vi "TimerDRV.vi"(8 "error in (no error)":errorcluster, 11 "TimerDRV in":refnum<class "TimerDRV.lvclass">) -> (0 "error out":errorcluster, 3 "TimerDRV out":refnum<class "TimerDRV.lvclass">)   [LabVIEW 2019, in "TimingDRV Engine.lvlib" / "TimerDRV.lvclass"]
uses:
  TimerDRV.lvclass
  TimerDRV.lvclass/TimerDRV.ctl
  <vilib>/Platform/TimedLoop/XDataNode/timing_clust.ctl
  <vilib>/Platform/TimedLoop/XDataNode/nitl_modes.ctl
  <vilib>/Platform/TimedLoop/XDataNode/wakeup.ctl
  TypeDefs/Command.ctl
  <vilib>/platform/TimedLoop/XDataNode/XDataNode.xnode
  <vilib>/Platform/TimedLoop/XDataNode/XDNodeRunTimeDep.lvlib
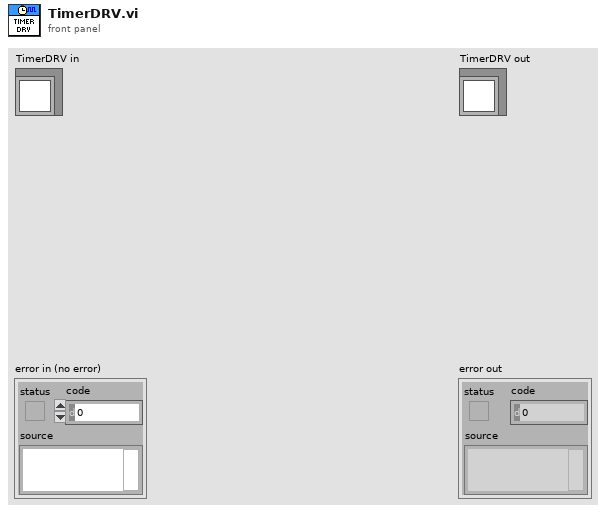
[diagram p1: front panel]
types:
  T1 = typedef "XDNodeRunTimeDep.lvlib/timing_clust.ctl" = cluster{"Expected End [f-1]":u64, "Actual End [f-1]":u64, "Finished Late? [f-1]":bool, "Expected End [i-1]":u64, "Actual End [i-1]":u64, "Finished Late? [i-1]":bool, "Expected Start [i]":u64, "Actual Start [i]":u64, "Expected Start [f]":u64, "Actual Start [f]":u64, "Source Name":string, "Structure Name":string, "Period":i64, "Deadline":i64, "Offset":i64, "Start":i64, "Priority":i32, "Timeout":i32, "Mode":T2, "Wakeup Reason":T3, "Error":errorcluster, "Source Type":string, "Secondary Source Type":string, "Global End Time":u64, "Global Start Time":u64, "Frame Duration":u64, "Iteration Duration":u64, "Assigned CPU":i32, "I/O Scan Engine Mode":u32}
  T2 = typedef "XDNodeRunTimeDep.lvlib/nitl_modes.ctl" = enum32{"No Change", "Process missed periods, maintain original phase", "Discard missed periods, maintain original phase", "Process missed periods, ignore original phase", "Discard missed periods, ignore original phase"}
  T3 = typedef "XDNodeRunTimeDep.lvlib/wakeup.ctl" = enum32{"Normal", "Aborted", "Asynchronous wakeup", "Timing source error", "Timed loop error", "Timeout"}
  T4 = typedef "TimingDRV Engine.lvlib/TimerDRV.lvclass/Command.ctl" = enum16{"Shutdown", "Update Execution Frequency", "Initialize"}
  T5 = typedef "TimingDRV Engine.lvlib/TimerDRV.lvclass/Target Type.ctl" = enum16{"PharLap", "VxWorks", "Windows", "Linux_32_ARM", "Linux_x64"}
  T6 = typedef "TimingDRV Engine.lvlib/TimerDRV.lvclass/Command Package.ctl" = cluster{"Command":T4, "Command Data":variant}
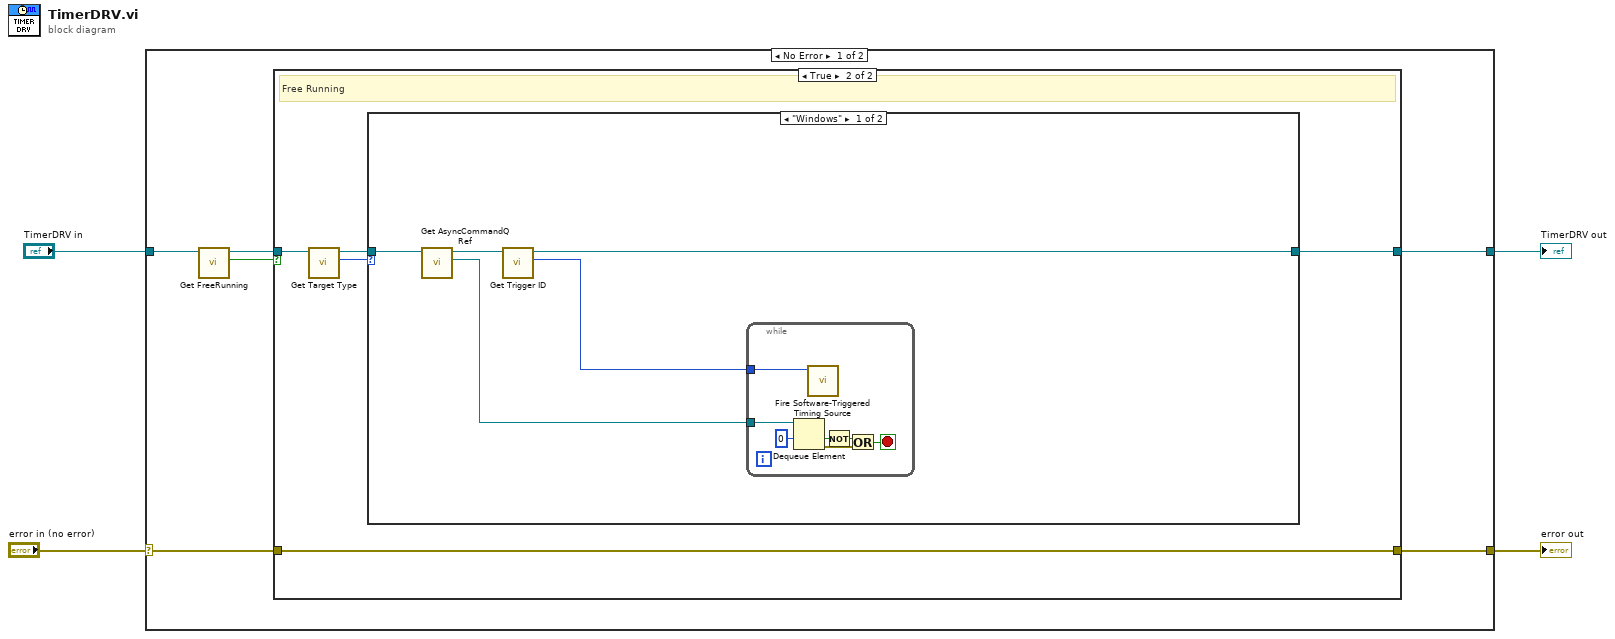
[diagram p0: block diagram]
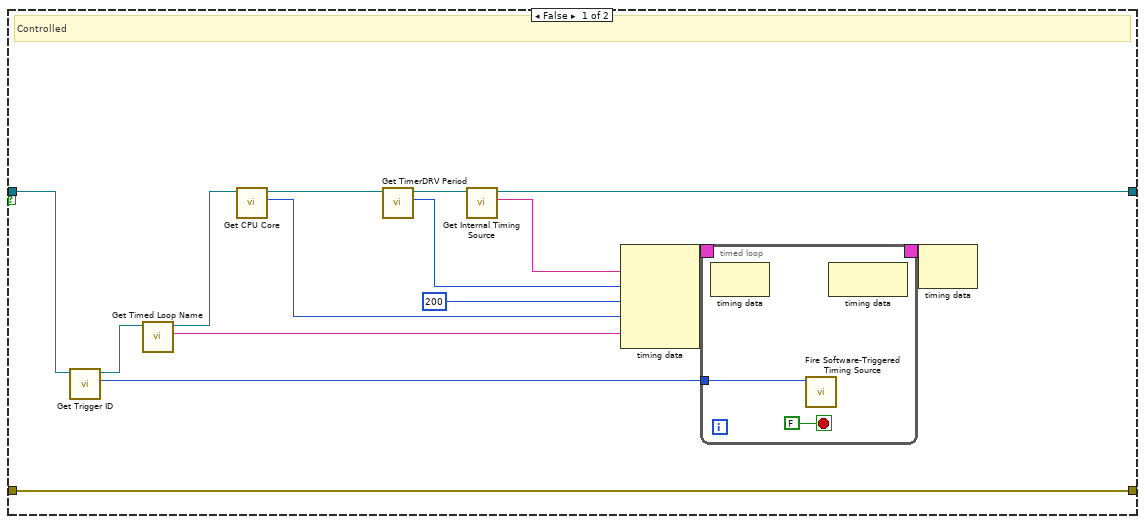
[diagram p2: hidden frame]
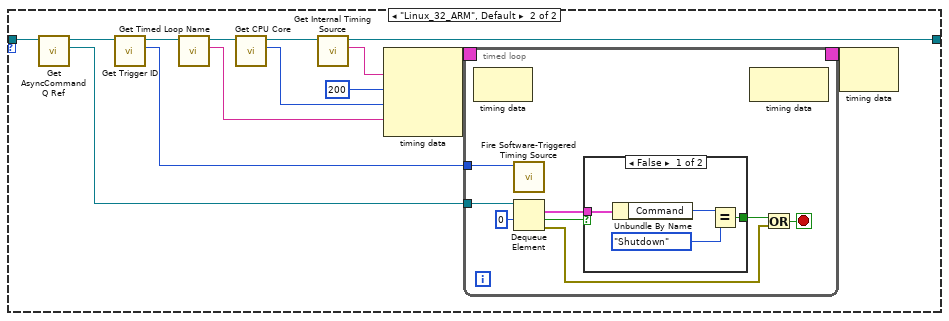
[diagram p3: hidden frame]
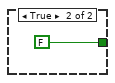
[diagram p4: hidden frame]
diagram:
  n1 = case shown="No Error" "error in (no error)" {
    selector: "error in (no error)" -> [w6 w92]
    tunnel: [w5 w92] -> w3
    tunnel: [w10 w91] -> w1
    tunnel: "TimerDRV in" -> [w9 w91]
    frame No Error {
      n2 = call "Get FreeRunning.vi"("TimerDRV in"=w9) -> ("FreeRunning"=w7:bool, "TimerDRV out"=w8:refnum<class "TimerDRV.lvclass">)  [unwired: 9 in]
      n3 = case shown="True" w7 {
        tunnel: [w18 w39] -> w10
        tunnel: w8 -> [w12 w42]
        tunnel: w6 -> [w11 w38]
        tunnel: [w11 w38] -> w5
        frame False {
          # "Controlled"
          n4 = call "Get Trigger ID.vi"("TimerDRV in"=w12) -> ("Trigger ID"=w16:u8, "TimerDRV out"=w15:refnum<class "TimerDRV.lvclass">)  [unwired: 9 in]
          n5 = call "Get Timed Loop Name.vi"("TimerDRV in"=w15) -> ("Timed Loop Name"=w14:string, "TimerDRV out"=w13:refnum<class "TimerDRV.lvclass">)  [unwired: 9 in]
          n6 = call "Get CPU Core.vi"("TimerDRV in"=w13) -> ("CPU Core"=w19:i32, "TimerDRV out"=w20:refnum<class "TimerDRV.lvclass">)  [unwired: 9 in]
          n7 = call "Get TimerDRV Period.vi"("TimerDRV in"=w20) -> ("TimerDRV Period"=w21:i64, "TimerDRV out"=w23:refnum<class "TimerDRV.lvclass">)  [unwired: 9 in]
          n8 = call "Get Internal Timing Source.vi"("TimerDRV in"=w23) -> ("Internal Timing Source"=w22:string, "TimerDRV out"=w18:refnum<class "TimerDRV.lvclass">)  [unwired: 9 in]
          n9 = node-c288(w22, w21, 200 ("Priority"), w19, w14) -> (w25:T1)
          n10 = timed-loop {
            timing: w25 -> [_]
            timing-out: [_] -> w24
            tunnel: w16 -> [w27]
            stop <- FALSE stop-if-true
            n11 = node-c288() -> ()  [unwired: 1 in, 1 out]
            n12 = call <vilib>:"Fire Software-Triggered Timing Source.vi"("trigger ID"=w27) -> ()  [unwired: 9 in, 2 out]
            n13 = node-c288() -> ()  [unwired: 1 in, 1 out]
          }
          n14 = node-c288(w24) -> ()  [unwired: 1 out]
        }
        frame True {
          # "Free Running"
          n15 = call "Get Target Type.vi"("TimerDRV in"=w42) -> ("Target Type"=w41:T5, "TimerDRV out"=w40:refnum<class "TimerDRV.lvclass">)  [unwired: 9 in]
          n16 = case shown="\"Windows\"" w41 {
            tunnel: w40 -> [w46 w67]
            tunnel: [w43 w55] -> w39
            frame "Windows" {
              n17 = call "Get AsyncCommandQ Ref.vi"("TimerDRV in"=w46) -> ("AsyncCommandQ"=w44:refnum<queue>, "TimerDRV out"=w45:refnum<class "TimerDRV.lvclass">)  [unwired: 9 in]
              n18 = call "Get Trigger ID.vi"("TimerDRV in"=w45) -> ("Trigger ID"=w47:u8, "TimerDRV out"=w43:refnum<class "TimerDRV.lvclass">)  [unwired: 9 in]
              n19 = while {
                tunnel: w47 -> [w54]
                tunnel: w44 -> [w53]
                stop <- w51 stop-if-true
                n20 = Dequeue Element(queue=w53, timeout in ms (-1)=0) -> (timed out?=w49:bool, error out=w50:errorcluster)  [unwired: 1 in, 2 out]
                n21 = call <vilib>:"Fire Software-Triggered Timing Source.vi"("trigger ID"=w54) -> ()  [unwired: 9 in, 2 out]
                n22 = Not(x=w49) -> (.not. x?=w48:bool)
                n23 = Or(x=w48, y=w50) -> (x .or. y?=w51:bool)
              }
            }
            frame "Linux_32_ARM", Default {
              n24 = call "Get AsyncCommandQ Ref.vi"("TimerDRV in"=w67) -> ("AsyncCommandQ"=w65:refnum<queue>, "TimerDRV out"=w66:refnum<class "TimerDRV.lvclass">)  [unwired: 9 in]
              n25 = call "Get Trigger ID.vi"("TimerDRV in"=w66) -> ("Trigger ID"=w68:u8, "TimerDRV out"=w62:refnum<class "TimerDRV.lvclass">)  [unwired: 9 in]
              n26 = call "Get Timed Loop Name.vi"("TimerDRV in"=w62) -> ("Timed Loop Name"=w60:string, "TimerDRV out"=w59:refnum<class "TimerDRV.lvclass">)  [unwired: 9 in]
              n27 = call "Get CPU Core.vi"("TimerDRV in"=w59) -> ("CPU Core"=w58:i32, "TimerDRV out"=w56:refnum<class "TimerDRV.lvclass">)  [unwired: 9 in]
              n28 = call "Get Internal Timing Source.vi"("TimerDRV in"=w56) -> ("Internal Timing Source"=w61:string, "TimerDRV out"=w55:refnum<class "TimerDRV.lvclass">)  [unwired: 9 in]
              n29 = node-c288(w61, 200 ("Priority"), w58, w60) -> (w64:T1)
              n30 = timed-loop {
                tunnel: w68 -> [w76]
                tunnel: w65 -> [w75]
                timing: w64 -> [_]
                timing-out: [_] -> w63
                stop <- w70 stop-if-true
                n31 = node-c288() -> ()  [unwired: 1 in, 1 out]
                n32 = call <vilib>:"Fire Software-Triggered Timing Source.vi"("trigger ID"=w76) -> ()  [unwired: 9 in, 2 out]
                n33 = Dequeue Element(queue=w75, timeout in ms (-1)=0) -> (element=w72:T6, timed out?=w73:bool, error out=w69:errorcluster)  [unwired: 1 in, 1 out]
                n34 = case shown="False" w73 {
                  tunnel: w72 -> [w82 _]
                  tunnel: [w79 FALSE] -> w71
                  frame False {
                    n35 = Unbundle By Name(w82) -> ("Command"=w81:T4)
                    n36 = Equal?(x=w81, y=Command."Shutdown") -> (x = y?=w79:bool)
                  }
                  frame True {
                  }
                }
                n37 = node-c288() -> ()  [unwired: 1 in, 1 out]
                n38 = Or(x=w71, y=w69) -> (x .or. y?=w70:bool)
              }
              n39 = node-c288(w63) -> ()  [unwired: 1 out]
            }
          }
        }
      }
    }
    frame Error {
    }
  }
  "error out" <- w3
  "TimerDRV out" <- w1
